vi "Write Calibration Data Array.vi"(5 "Port (1)":i32=1, 7 "Channel (1)":i32=1, 8 "error in (no error)":errorcluster, 9 "Calibration Data Array (0)":dbl[](array[numeric]), 11 "VISA resource name":refnum<visa-resource-name>) -> (0 "error out":errorcluster, 3 "VISA resource name out":refnum<visa-resource-name>)   [LabVIEW 2011, in "Agilent ENA Series.lvlib"]
doc: "For selected port of selected channel, sets the power calibration data array."
uses:
  Agilent ENA Series.lvlib
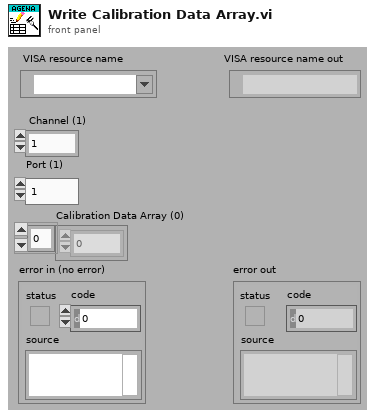
[diagram p1: front panel]
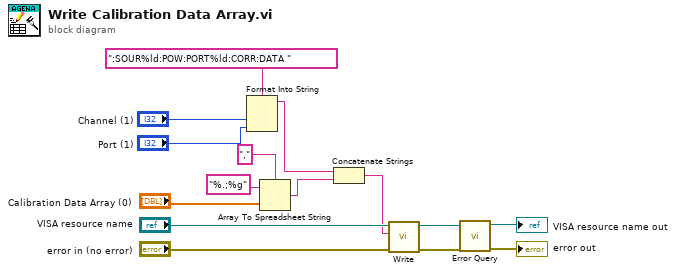
[diagram p0: block diagram]
diagram:
  n1 = Format Into String(format string=":SOUR%ld:POW:PORT%ld:CORR:DATA ", "Channel (1)", "Port (1)") -> (resulting string=w7:string)  [unwired: 2 in, 1 out]
  n2 = Array To Spreadsheet String(delimiter (Tab)=",", array="Calibration Data Array (0)", 3:"%.;%g" ("format string")) -> (spreadsheet string=w6:string)
  n3 = Concatenate Strings(w7, w6) -> (w5:string)
  n4 = call "Write.vi"("error in (no error)"="error in (no error)", "String ()"=w5, "VISA resource name"="VISA resource name") -> ("error out"=w3:errorcluster, "VISA resource name out"=w4:refnum<visa-resource-name>)  [unwired: 6 in, 1 out]
  n5 = call "Error Query.vi"("error in (no error)"=w3, "VISA resource name"=w4) -> ("error out"=→"error out":errorcluster, "VISA resource name out"=→"VISA resource name out":refnum<visa-resource-name>)  [unwired: 6 in, 2 out]
